vi "ao_voltage.vi"(4 "lower limit":dbl=-1.5, 6 "upper limit":dbl=1.5, 7 "hold (ms)":u32, 8 "error in":errorcluster, 10 "value":dbl) -> (0 "error out":errorcluster, 2 "value out":dbl format="%#_13g")   [LabVIEW 2017]
panel:
  in  "device":tag="Dev1"
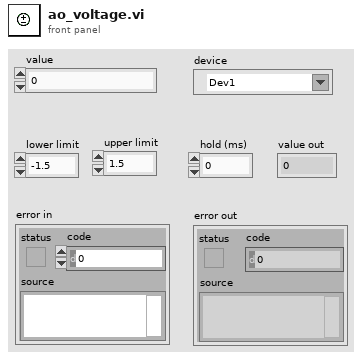
[diagram p1: front panel]
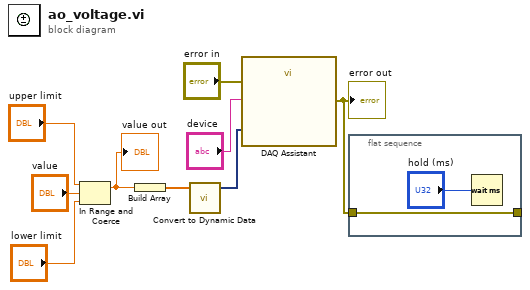
[diagram p0: block diagram]
diagram:
  n1 = In Range and Coerce(upper limit="upper limit", x="value", lower limit="lower limit") -> (coerced(x)=w3:dbl)  [unwired: 1 out]
  "value out" <- w3
  n2 = Build Array(w3) -> (w8:dbl[])
  n3 = call "Convert to Dynamic Data"("Array"=w8) -> ("Dynamic Data Type"=w9:dynamicdata)  [unwired: 3 in]
  n4 = call "DAQ Assistant"("data"=w9, "error in"="error in", "device name"="device") -> ("error out"=w4:errorcluster)  [unwired: 15 in, 1 out]
  "error out" <- w4
  n5 = flat-sequence {
    tunnel: [w10] -> _
    tunnel: w4 -> [w10]
    frame #0 {
      n6 = Wait (ms)(milliseconds to wait="hold (ms)") -> ()  [unwired: 1 out]
    }
  }
